vi "Program CT Device.vi"(8 "error in (no error)":errorcluster, 11 "CTT Programming Test in":refnum<class "CTT Programming Test.lvclass">) -> (0 "error out":errorcluster, 2 "Passed":bool, 3 "CTT Programming Test out":refnum<class "CTT Programming Test.lvclass">)   [LabVIEW 2015, in "CTT Programming Test.lvclass"]
uses:
  CTT Programming Test.lvclass
  <vilib>/Cree, Inc/Cree Test Framework/Core Launcher/Core Manager Methods -- Enum.ctl
  Classes/Programmer/Atmel e-ICE/Class/Atmel e-ICE.lvclass
  Classes/Programmer/Atmel ICE/Atmel ICE.lvlib
  <vilib>/Cree, Inc/Cree Test Framework/Classes/Data/Data Repo/Class/Data Repo.lvclass
  <vilib>/Cree, Inc/Cree Test Framework/Core Launcher/Core Launcher.lvlib
  Classes/Application/Class/Application.lvclass
  Classes/Test Recipe/Class/Test Recipe.lvclass
  Test Class/Test Class.lvclass
  <vilib>/Cree, Inc/Cree Test Framework/Classes/Base Objects/Base Class/Base Class/Base Class.lvclass
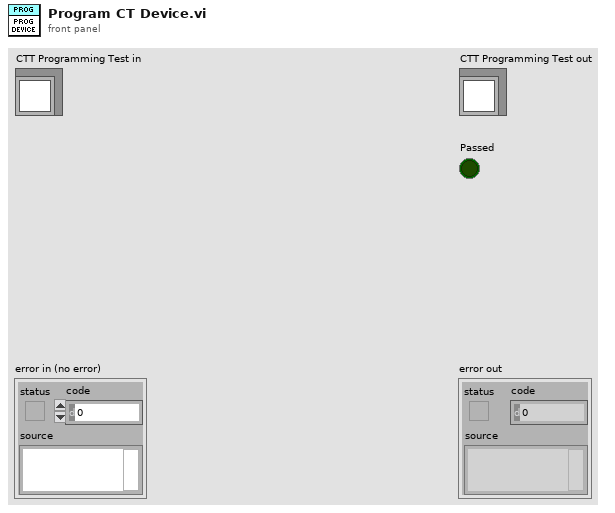
[diagram p1: front panel]
types:
  T1 = typedef "Core Launcher.lvlib/Core Manager Methods -- Enum.ctl" = enum16{"Spawn Objects", "Get Objects", "Destroy Objects"}
  T2 = typedef "Application.lvlib/App Properties.lvclass/Class Properties -- Cluster.ctl" = cluster{"UUT Info":T3[], "Test Information":refnum<vi>, "Test Complete Event":refnum<user-event>, "Shop Floor System":refnum<class "Shop Floor System.lvclass">, "Gold Board":refnum<class "Golden Board.lvclass">, "Test Recipe":refnum<class "Test Recipe.lvclass">, "Instruments":refnum<class "Instrument.lvclass">[], "Mode":T4, "Test Results":cluster{"Pass":bool[], "Fail Codes":string[]}, "Station Config":refnum<class "Station Config.lvclass">}
  T3 = typedef "Application.lvlib/App Properties.lvclass/UUT Reference -- Cluster.ctl" = cluster{"Serial Number Reference":refnum<vi>, "Status Message Reference":refnum<vi>}
  T4 = typedef "Application.lvlib/Application.lvclass/Op Mode -- Enum.ctl" = u16
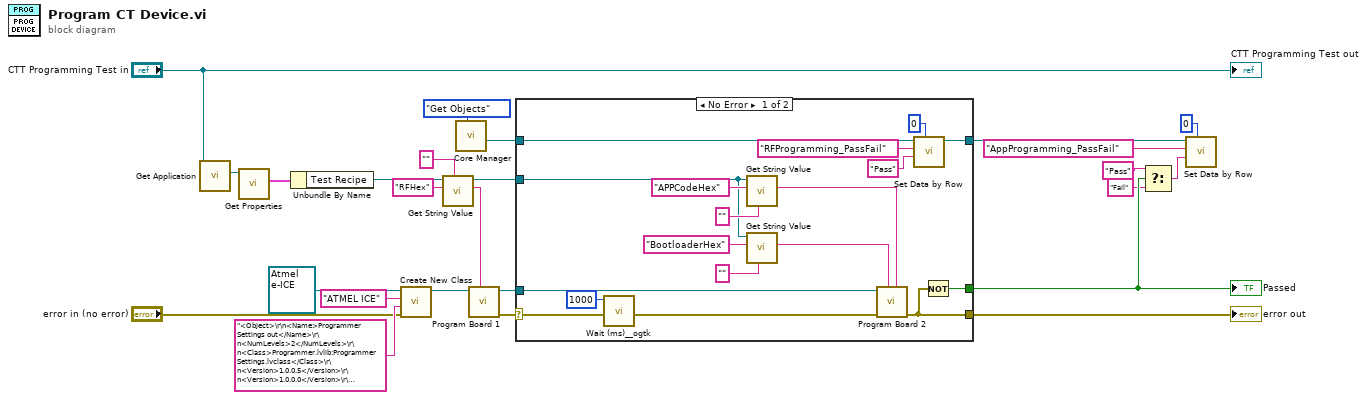
[diagram p0: block diagram]
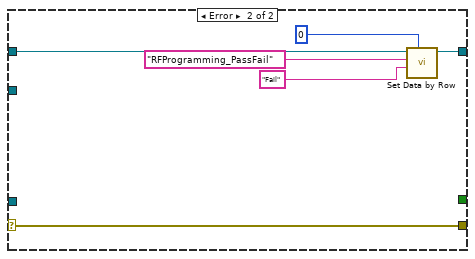
[diagram p2: hidden frame]
diagram:
  n1 = call "Get Application.vi"("Test Class in"="CTT Programming Test in") -> ("Application.lvlib:Application.lvclass"=w12:refnum<class "Application.lvclass">)  [unwired: 9 in, 1 out]
  n2 = call "Get Properties.vi"("Acrobat Template in"=w12) -> ("Class Properties"=w23:T2)  [unwired: 8 in, 2 out]
  n3 = Unbundle By Name(w23) -> ("Test Recipe"=w11:refnum<class "Test Recipe.lvclass">)
  n4 = call <vilib>:"Create New Class.vi"("error in (no error)"="error in (no error)", "Configuration"="<Object>\r\n<Name>Programmer Settings out</Name>\r\n<NumLevels>2</NumLevels>\r\n<Class>Programmer.lvlib:Programmer Settings.lvclass</Class>\r\n<Version>1.0.0.5</Version>\r\n<Version>1.0.0.0</Version>\r\n<Cluster>\r\n</Cluster>\r\n<Cluster>\r\n<Name>Programmer Settings.lvclass</Name>\r\n<NumElts>1</NumElts>\r\n<Cluster>\r\n<Name>Class Settings</Name>\r\n<NumElts>12</NumElts>\r\n<String>\r\n<Name>Local Path</Name>\r\n<Val>C:\\Programmer</Val>\r\n</String>\r\n<String>\r\n<Name>Network Path</Name>\r\n<Val>W:\\Programmer</Val>\r\n</String>\r\n<Boolean>\r\n<Name>Local Enable</Name>\r\n<Val>1</Val>\r\n</Boolean>\r\n<String>\r\n<Name>System Version</Name>\r\n<Val>v1.5</Val>\r\n</String>\r\n<String>\r\n<Name>Flash Hex File</Name>\r\n<Val></Val>\r\n</String>\r\n<String>\r\n<Name>Lockbits Hex File</Name>\r\n<Val></Val>\r\n</String>\r\n<String>\r\n<Name>Fuse Hex File</Name>\r\n<Val></Val>\r\n</String>\r\n<String>\r\n<Name>Revision</Name>\r\n<Val>1.05.207</Val>\r\n</String>\r\n<String>\r\n<Name>Chip Type</Name>\r\n<Val></Val>\r\n</String>\r\n<String>\r\n<Name>JTAG Serial Number</Name>\r\n<Val></Val>\r\n</String>\r\n<String>\r\n<Name>JTAG Clock</Name>\r\n<Val>6mhz</Val>\r\n</String>\r\n<I32>\r\n<Name>Number of Retries</Name>\r\n<Val>2</Val>\r\n</I32>\r\n</Cluster>\r\n</Cluster>\r\n</Object>\r\n" ("xml string"), "Name"="ATMEL ICE", "Base Class in"=refnum<class "Atmel e-ICE.lvclass"> refnum ("Atmel e-ICE.lvlib:Atmel e-ICE.lvclass")) -> ("Base Class out"=w2:refnum<class "Atmel e-ICE.lvclass">)  [unwired: 6 in, 1 out]
  n5 = call "Get String Value.vi"("Default Value"="", "Name"="RFHex", "Test Recipe in"=w11) -> ("Value"=w8:string, "Test Recipe out"=w7:refnum<class "Test Recipe.lvclass">)  [unwired: 6 in, 1 out]
  n6 = call <vilib>:"Core Manager.vi"("Method"=Core_Manager_Methods_--_Enum."Get Objects") -> ("Data Repo"=w22:refnum<class "Data Repo.lvclass">)  [unwired: 7 in, 3 out]
  n7 = call "Program Board 1.vi"("RF File"=w8, "Programmer"=w2) -> ("error out"=w20:errorcluster, "Programmer"=w19:refnum<class "Atmel e-ICE.lvclass">)  [unwired: 8 in]
  n8 = case shown="No Error" w20 {
    selector: w20 -> [w28 w49]
    tunnel: w19 -> [w43 _]
    tunnel: [w42 _] -> w24
    tunnel: [w41 w49] -> w1
    tunnel: w22 -> [w40 w46]
    tunnel: [w36 w44] -> w16
    tunnel: w7 -> [w30 _]
    frame No Error {
      n9 = call <userlib>:"Wait (ms)__ogtk.vi"("error in (no error)"=w28, "milliseconds to wait"=u32 1000) -> ("error out"=w26:errorcluster)  [unwired: 8 in, 1 out]
      n10 = call "Get String Value.vi"("Default Value"="", "Name"="APPCodeHex", "Test Recipe in"=w30) -> ("Value"=w33:string)  [unwired: 6 in, 2 out]
      n11 = call "Get String Value.vi"("Default Value"="", "Name"="BootloaderHex", "Test Recipe in"=w30) -> ("Value"=w29:string)  [unwired: 6 in, 2 out]
      n12 = call "Program Board 2.vi"("APP Code Hex"=w33, "Bootloader Hex"=w29, "error in (no error)"=w26, "Programmer"=w43) -> ("error out"=w41:errorcluster)  [unwired: 6 in, 1 out]
      n13 = call <vilib>:"Set Data by Row.vi"("Row"=0, "Value"="Pass", "Header"="RFProgramming_PassFail" ("Placeholder"), "Acrobat Template in"=w40) -> ("Acrobat Template out"=w36:refnum<class "Data Repo.lvclass">)  [unwired: 6 in, 1 out]
      n14 = Not(x=w41) -> (.not. x?=w42:bool)
    }
    frame Error {
      n15 = call <vilib>:"Set Data by Row.vi"("Row"=0, "Value"="Fail", "Header"="RFProgramming_PassFail" ("Placeholder"), "Acrobat Template in"=w46) -> ("Acrobat Template out"=w44:refnum<class "Data Repo.lvclass">)  [unwired: 6 in, 1 out]
    }
  }
  "error out" <- w1
  "Passed" <- w24
  n16 = Select(t="Pass" ("Value"), s=w24, f="Fail" ("Value")) -> (s? t:f=w13:string)
  n17 = call <vilib>:"Set Data by Row.vi"("Row"=0, "Value"=w13, "Header"="AppProgramming_PassFail" ("Placeholder"), "Acrobat Template in"=w16) -> ()  [unwired: 6 in, 2 out]
  "CTT Programming Test out" <- "CTT Programming Test in"
